vi "RegWriteExtLong UnitTest.vi"() -> ()   [LabVIEW 2018]
uses:
  Downloads/MIPI RFFE API/Controls/RFFE Commands Type Def.ctl
  Downloads/MIPI RFFE API/Controls/Write Data Strict Type Def.ctl
  Command/RFFE Command.lvclass
  RegWriteExtLong/RFFE RegWriteExtLong Command.lvclass
  C:/Users/semoore/Projects/mipi-rffe-labview-oop/Command/RFFE Command.lvclass
panel:
  out "arrays same size?":bool
  out "data equal?":bool
  out "error in (no error) 2":errorcluster
  in  "error in (no error)":errorcluster
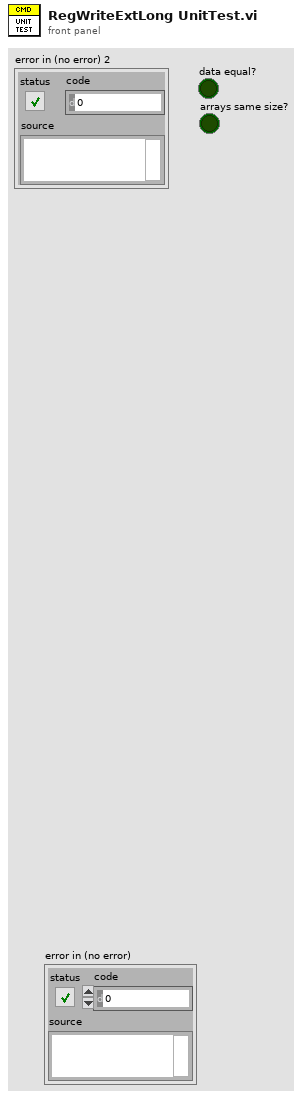
[diagram p1: front panel]
types:
  T1 = typedef "Write Data Strict Type Def.ctl" = cluster{"slave address":u8, "register address":u16, "register data (write)":u8[], "byte count":u8}
  T2 = typedef "RFFE Commands Type Def.ctl" = enum16{"Reg0Write", "RegWrite", "RegRead", "RegReadHR", "RegWriteExt", "RegReadExt", "RegReadExtHR", "RegWriteExtLong", "RegReadExtLong", "RegReadExtLongHR"}
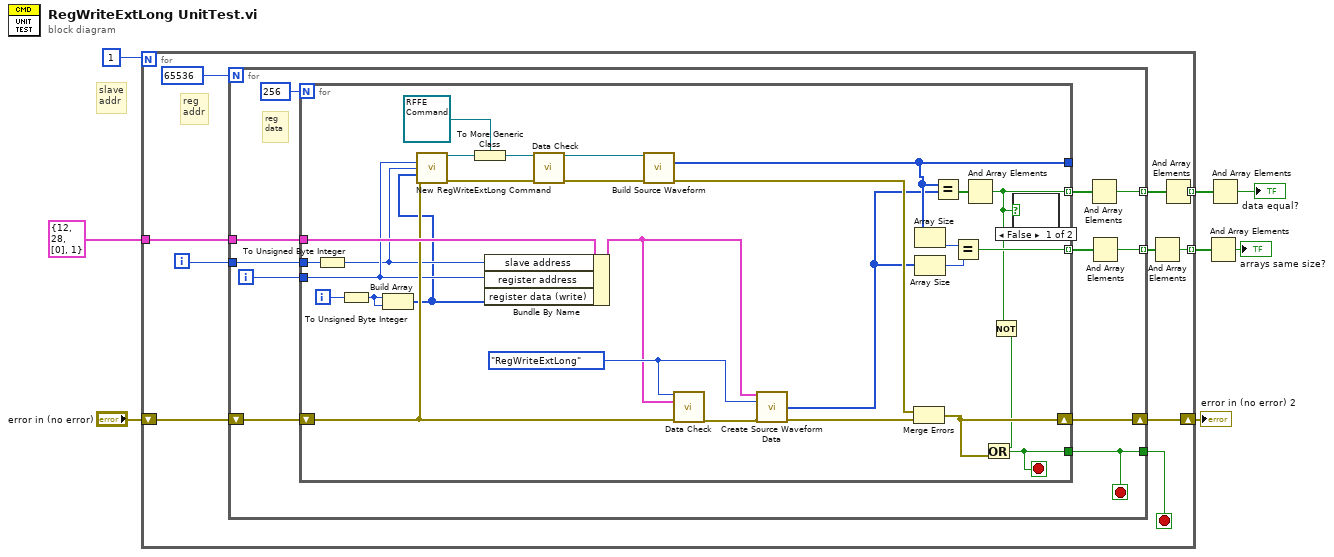
[diagram p0: block diagram]
diagram:
  # "slave\naddr"
  n1 = for {
    N: 1 -> [_]
    tunnel: T1 {"slave address"=12, "register address"=28, "register data (write)"=[0], "byte count"=1} ("Register Data") -> [w17]
    shift-right: [w14] -> w5
    shift-left: "error in (no error)" -> [w18]
    tunnel: [w12] -> w4 mode=indexing
    tunnel: [w10] -> w2 mode=indexing
    i -> [w16]
    stop <- w9 stop-if-true
    # "reg\naddr"
    n2 = for {
      N: 65536 -> [_]
      tunnel: w17 -> [w28]
      tunnel: w16 -> [w25]
      shift-right: [w24] -> w14
      shift-left: w18 -> [w29]
      tunnel: [w22] -> w13 mode=indexing
      tunnel: [w20] -> w11 mode=indexing
      tunnel: [w19] -> w9
      i -> [w26]
      stop <- w19 stop-if-true
      # "reg\ndata"
      n3 = for {
        N: 256 -> [_]
        tunnel: w28 -> [w56]
        tunnel: [w34] -> _
        tunnel: w26 -> [w39]
        tunnel: w25 -> [w45]
        shift-right: [w49] -> w24
        shift-left: w29 -> [w46]
        tunnel: [w32] -> w23 mode=indexing
        tunnel: [w37] -> w21 mode=indexing
        tunnel: [w31] -> w19
        i -> [w44]
        stop <- w31 stop-if-true
        w58 = RFFE_Commands_Type_Def."RegWriteExtLong" ("RFFE command")
        n4 = To Unsigned Byte Integer(number=w45) -> (unsigned 8bit integer=w38:u8)
        n5 = To Unsigned Byte Integer(number=w44) -> (unsigned 8bit integer=w36:u8)
        n6 = Build Array(w36, w36) -> (w35:u8[])
        n7 = call "New RegWriteExtLong Command.vi"("Register Address"=w39, "Slave Address"=w38, "Register Data"=w35, "error in (no error)"=w46) -> ("RFFE RegWriteExt Command out"=w52:refnum<class "RFFE RegWriteExtLong Command.lvclass">, "error out"=w53:errorcluster)  [unwired: 10 in]
        n8 = To More Generic Class(target class=refnum<class "RFFE Command.lvclass"> refnum ("RFFE Commands.lvlib:RFFE Command.lvclass"), reference=w52) -> (generic class reference=w41:refnum<class "RFFE Command.lvclass">)
        n9 = Bundle By Name(cluster=w56, "slave address"=w38, "register address"=w39, "register data (write)"=w35) -> (w55:T1)
        n10 = call-dynamic "Data Check.vi"("RFFE Command in"=w41, "error in (no error)"=w53) -> ("RFFE Command out"=w51:refnum<class "RFFE Command.lvclass">, "error out"=w54:errorcluster)  [unwired: 12 in]
        n11 = call-dynamic "Build Source Waveform.vi"("RFFE Command in"=w51, "error in (no error)"=w54) -> ("Source Waveform"=w34:u32[], "error out"=w48:errorcluster)  [unwired: 11 in, 1 out]
        n12 = call "Data Check.vi"("RFFE command"=w58, "Register Data"=w55, "error in"=w46) -> ("error out"=w57:errorcluster)  [unwired: 12 in]
        n13 = call "Create Source Waveform Data.vi"("Register Data"=w55, "RFFE command"=w58, "error in"=w57) -> ("RFFEWrite source waveform data array"=w33:u32[], "error out"=w50:errorcluster)  [unwired: 10 in, 1 out]
        n14 = Merge Errors(w48, w50) -> (w49:errorcluster)
        n15 = Array Size(array=w34) -> (size(s)=w43:i32)
        n16 = Array Size(array=w33) -> (size(s)=w42:i32)
        n17 = Equal?(x=w34, y=w33) -> (x = y?=w47:bool[])
        n18 = Equal?(x=w43, y=w42) -> (x = y?=w37:bool)
        n19 = And Array Elements(Boolean array=w47) -> (logical AND=w32:bool)
        n20 = Not(x=w32) -> (.not. x?=w30:bool)
        n21 = Or(x=w30, y=w49) -> (x .or. y?=w31:bool)
        n22 = case shown="False" w32 {
          frame False {
          }
          frame True {
          }
        }
      }
      n23 = And Array Elements(Boolean array=w23) -> (logical AND=w22:bool)
      n24 = And Array Elements(Boolean array=w21) -> (logical AND=w20:bool)
    }
    n25 = And Array Elements(Boolean array=w11) -> (logical AND=w10:bool)
    n26 = And Array Elements(Boolean array=w13) -> (logical AND=w12:bool)
  }
  "error in (no error) 2" <- w5
  n27 = And Array Elements(Boolean array=w2) -> (logical AND=→"arrays same size?":bool)
  n28 = And Array Elements(Boolean array=w4) -> (logical AND=→"data equal?":bool)
